vi "temperaturesensorCalibration.vi"() -> ()   [LabVIEW 2022 SP3]
uses:
  <vilib>/DAQmx/read.llb/DAQmx Read (Analog DBL 1Chan 1Samp).vi
  <vilib>/DAQmx/create/channels.llb/DAQmx Create Channel (AI-Voltage-Basic).vi
  <vilib>/DAQmx/miscellaneous.llb/DAQmx Fill In Error Info.vi
panel:
  out "Numeric":dbl
  in  "physical channels":tag
  in  "stop":bool
  out "Meter":dbl(knob) scale=0.0..5.0
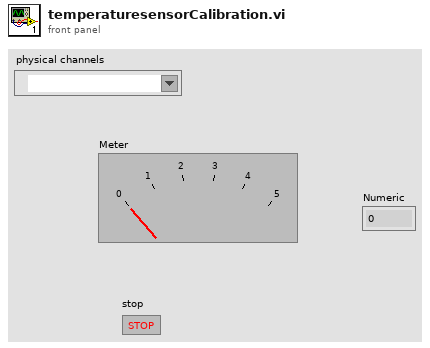
[diagram p1: front panel]
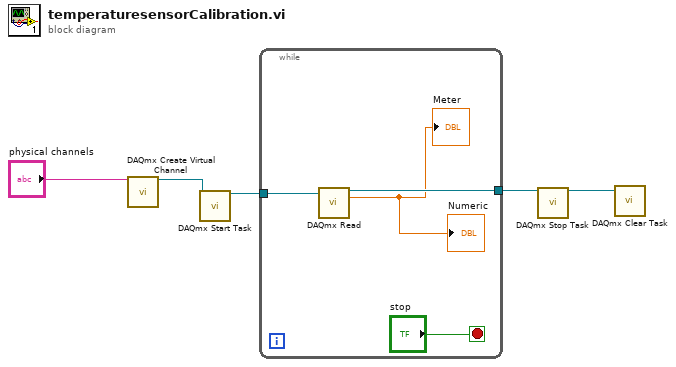
[diagram p0: block diagram]
diagram:
  n1 = call-poly <vilib>:"DAQmx Create Virtual Channel.vi"("physical channels"="physical channels") -> ("task out"=w5:refnum<k21>)  [unwired: 13 in, 1 out]
  n2 = call <vilib>:"DAQmx Start Task.vi"("task/channels in"=w5) -> ("task out"=w2:refnum<k21>)  [unwired: 13 in, 1 out]
  n3 = while {
    tunnel: [w8] -> w3
    tunnel: w2 -> [w7]
    stop <- "stop" stop-if-true
    n4 = call-poly <vilib>:"DAQmx Read.vi"("task/channels in"=w7) -> ("task out"=w8:refnum<k21>, "data"=→"Meter" →"Numeric":dbl)  [unwired: 12 in, 1 out]
  }
  n5 = call <vilib>:"DAQmx Stop Task.vi"("task/channels in"=w3) -> ("task out"=w4:refnum<k21>)  [unwired: 13 in, 1 out]
  n6 = call <vilib>:"DAQmx Clear Task.vi"("task in"=w4) -> ()  [unwired: 14 in, 1 out]
